vi "Check File Permissions.vi"(8 "error out":errorcluster, 11 "appended path":path) -> (0 "error IO":errorcluster)   [LabVIEW 2010]
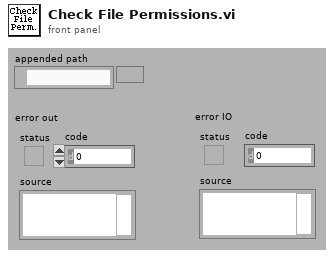
[diagram p1: front panel]
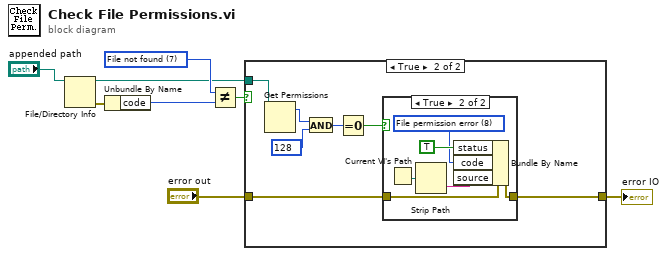
[diagram p0: block diagram]
diagram:
  w5 = 7 items=["No error", "Argument error", "Memory is full", "Out of zone", "End of file", "File already open", "Generic file I/O error", "File not found", "File permission error", "Disk is full", "Duplicate path", "Too many files open", "System feature not enabled", "Resource file not found", "Cannot add resource", "Resource not found", "Image not found", "Image memory error", "Pen does not exist", "Config type invalid", "Config token not found", "Config parse error", "Config memory error", "Bad external code format", "Bad external code offset", "External code not present", "Null window", "Destroy window error", "Null menu", "Print aborted", "Bad print record", "Print driver error", "Windows error during printing", "Memory error during printing", "Print dialog error", "Generic print error", "Invalid device refnum", "Device not found", "Device parameter error", "Device unit error", "Cannot open device", "Device call aborted", "Generic error", "Cancelled by user", "Object ID too low", "Object ID too high", "Object not in heap", "Unknown heap", "Unknown object (invalid DefProc)", "Unknown object (DefProc not in table)", "Message out of range", "Invalid (null) method", "Unknown message", "Manager call not supported", "Bad address", "Network operation in progress", "Network operation timed out", "Connection is busy", "Network attribute not supported", "Network error", "Address in use", "System out of memory", "Connection aborted", "Connection refused", "Not connected", "Already connected", "Connection closed", "Initialization error (interapplication manager)", "Bad occurrence", "Wait on unbound occurrence handler", "Occurrence queue overflow", "Datalog type conflict", "Unused", "Unrecognized type (interapplication manager)", "Memory corrupt", "Failed to make temporary DLL", "Old CIN version", "Drag socket not found", "Failed to load drop-object", "Failed to register OLE object", "Failed to release OLE object", "Format specifier type mismatch", "Unknown format specifier", "Too few format specifiers", "Too many format specifiers", "Scan failed", "Newer CIN version", "Error converting to variant", "Runtime menu error", "Password tampered", "Variant attribute not found", "Incompatible variant data type", "Event data is not available", "Event Store is not present", "Occurrence is not found", "Event Queue is not created", "Event info is not available", "Refnum passed is NULL", "Error retrieving Class GUID", "Error retrieving CoClass GUID", "Error retrieving TypeLib GUID.", "Bad built application magic bytes.", "Specific driver is different from the specific driver associated with the Logical Name.", "There is no session opened to the class driver.", "Max Error", "MAX - Error with config objects", "MAX - Error loading configuration", "MAX - Group not supported", "Singlecast connections can not send to multicast addresses.", "Multicast connections can not send to singlecast addresses.", "Specified IP address not in multicast address range.", "Attempt to write to read-only multicast connection.", "Attempt to read from write-only multicast connection.", "The buffer used to receive a datagram was smaller than the datagram itself"]
  n1 = File/Directory Info(path="appended path") -> (path out=w1:path, error out=w6:errorcluster)  [unwired: 1 in, 5 out]
  n2 = Unbundle By Name(w6) -> ("code"=w4:i32)
  n3 = Not Equal?(x=w5, y=w4) -> (x != y?=w3:bool)
  n4 = case shown="True" w3 {
    tunnel: "error out" -> [w9 w16]
    tunnel: [w9 w11] -> w2
    tunnel: w1 -> [_ w10]
    frame False {
    }
    frame True {
      n5 = Get Permissions(11:w10) -> (5:w14:i16)  [unwired: 1 in, 4 out]
      n6 = And(x=w14, y=128) -> (x .and. y?=w13:i32)
      n7 = Equal To 0?(x=w13) -> (x = 0?=w12:bool)
      n8 = case shown="True" w12 {
        tunnel: w16 -> [w17 w23]
        tunnel: [w17 w22] -> w11
        frame False {
        }
        frame True {
          w20 = u16 8 items=["No error", "Argument error", "Memory is full", "Out of zone", "End of file", "File already open", "Generic file I/O error", "File not found", "File permission error", "Disk is full", "Duplicate path", "Too many files open", "System feature not enabled", "Resource file not found", "Cannot add resource", "Resource not found", "Image not found", "Image memory error", "Pen does not exist", "Config type invalid", "Config token not found", "Config parse error", "Config memory error", "Bad external code format", "Bad external code offset", "External code not present", "Null window", "Destroy window error", "Null menu", "Print aborted", "Bad print record", "Print driver error", "Windows error during printing", "Memory error during printing", "Print dialog error", "Generic print error", "Invalid device refnum", "Device not found", "Device parameter error", "Device unit error", "Cannot open device", "Device call aborted", "Generic error", "Cancelled by user", "Object ID too low", "Object ID too high", "Object not in heap", "Unknown heap", "Unknown object (invalid DefProc)", "Unknown object (DefProc not in table)", "Message out of range", "Invalid (null) method", "Unknown message", "Manager call not supported", "Bad address", "Network operation in progress", "Network operation timed out", "Connection is busy", "Network attribute not supported", "Network error", "Address in use", "System out of memory", "Connection aborted", "Connection refused", "Not connected", "Already connected", "Connection closed", "Initialization error (interapplication manager)", "Bad occurrence", "Wait on unbound occurrence handler", "Occurrence queue overflow", "Datalog type conflict", "Unused", "Unrecognized type (interapplication manager)", "Memory corrupt", "Failed to make temporary DLL", "Old CIN version", "Drag socket not found", "Failed to load drop-object", "Failed to register OLE object", "Failed to release OLE object", "Format specifier type mismatch", "Unknown format specifier", "Too few format specifiers", "Too many format specifiers", "Scan failed", "Newer CIN version", "OLE Convert", "Runtime menu error", "Password tampered", "Unknown error code"]
          n9 = Current VI's Path() -> (path=w19:path)
          n10 = Strip Path(path=w19) -> (name=w18:string)  [unwired: 1 out]
          n11 = Bundle By Name(cluster=w23, "status"=TRUE, "code"=w20, "source"=w18) -> (w22:errorcluster)
        }
      }
    }
  }
  "error IO" <- w2
